vi "write_to_memory.vi"(2 "Column":i32, 3 "Row":i32, 4 "New element":u8, 5 "Memory Out":T1) -> (0 "Memory Out 2":T1)   [LabVIEW 2009]
uses:
  behaviors/occupancy grid memory typedef.ctl
  <vilib>/rvi/DataTransferAndStorage/Container/XNode/niFpgaContainer.xnode
  <vilib>/rvi/DataTransferAndStorage/Container/Common/niFpgaContainerExecOnDevCompGetState.vi
  <vilib>/rvi/DataTransferAndStorage/Container/Common/niFpgaContainerMetaDataKey.ctl
  <vilib>/rvi/Memory/Memory_Emulation/nirvimemoryEmulationManagerCache_GetValue.vi
  <vilib>/rvi/Memory/Memory_Emulation/nirvimemoryEmulationManagerCache_InsertValue.vi
  <vilib>/rvi/FIFO/Fifo_Resource/nirvififoUniquifyingName.vi
  <vilib>/Utility/error.llb/Clear Errors.vi
  <vilib>/rvi/Memory/Memory_Emulation/nirvimemoryEmulationManagerCache_SetValue.vi
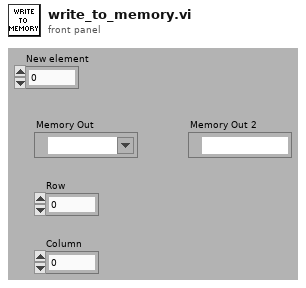
[diagram p1: front panel]
types:
  T1 = typedef "occupancy grid memory typedef.ctl" = refnum<k21>
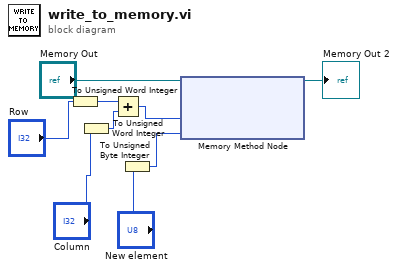
[diagram p0: block diagram]
diagram:
  n1 = To Unsigned Word Integer(number="Row") -> (unsigned 16bit integer=w7:u16)
  n2 = To Unsigned Word Integer(number="Column") -> (unsigned 16bit integer=w8:u16)
  n3 = Add(x=w7, y=w8) -> (x+y=w9:u16)
  n4 = To Unsigned Byte Integer(number="New element") -> (unsigned 8bit integer=w4:u8)
  n5 = xnode ("Memory Method Node")("Address"=w9, "Data"=w4, "Memory In"="Memory Out") -> ("Memory Out"=→"Memory Out 2":T1)
